vi "Configure Math (Add).vi"(0 "VISA resource name":refnum<visa-resource-name>, 2 "Vertical Scale (2)":dbl=2.0, 5 "Channel A (1: Channel 1)":i32(ring)=1 items=["Channel 1"=1, "Channel 2"=2, "Channel 3"=3, "Channel 4"=4], 7 "Channel B (2: Channel 2)":i32(ring)=2 items=["Channel 1"=1, "Channel 2"=2, "Channel 3"=3, "Channel 4"=4], 9 "Enable Invert Display (F: Disable)":bool, 11 "error in (no error)":errorcluster, 12 "Vertical Offset (0)":dbl) -> (4 "VISA resource name out":refnum<visa-resource-name>, 15 "error out":errorcluster)   [LabVIEW 2015, in "ZhiYuan ZDS Series for TCP.lvlib"]
doc: "Configures the setting for math operation with two operands."
uses:
  ZhiYuan ZDS Series for TCP.lvlib
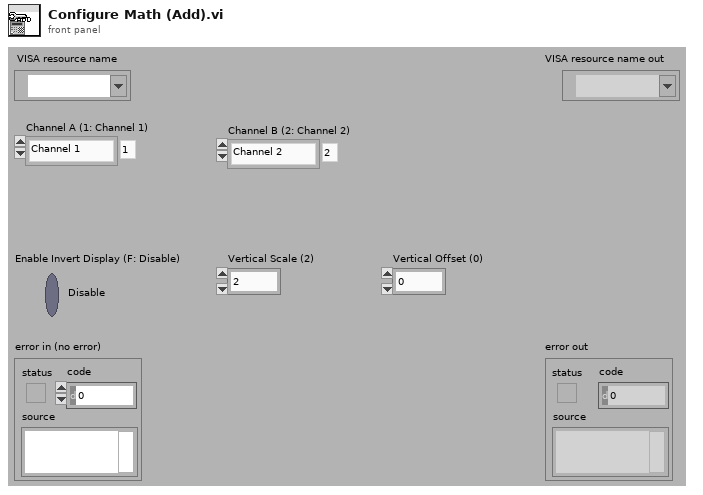
[diagram p1: front panel]
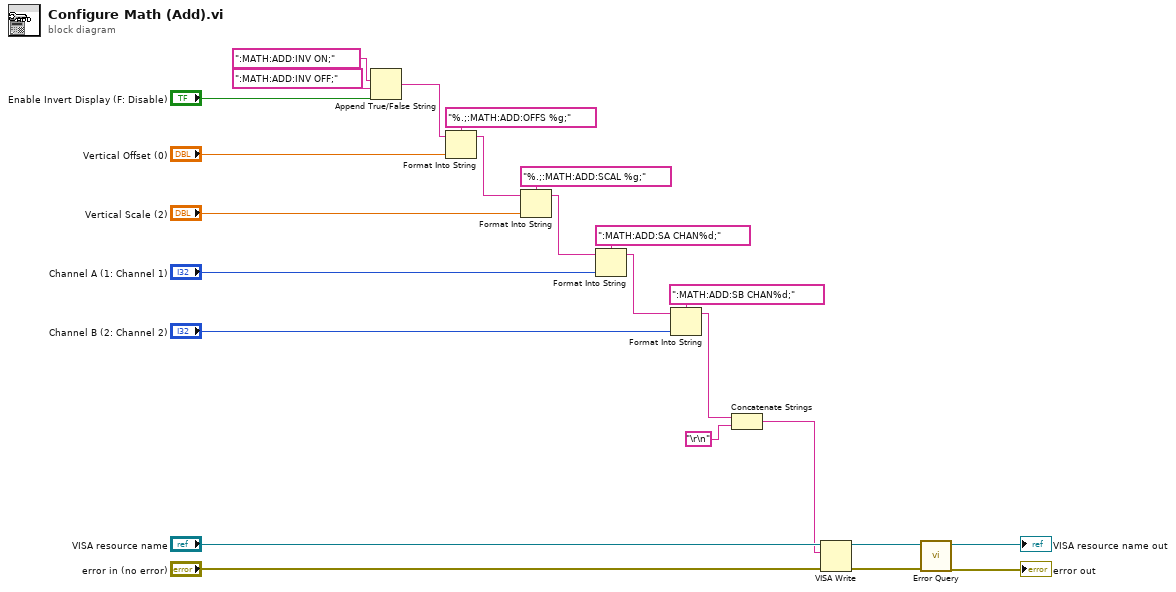
[diagram p0: block diagram]
diagram:
  n1 = Append True/False String(1:"Enable Invert Display (F: Disable)", 2:":MATH:ADD:INV OFF;", 3:":MATH:ADD:INV ON;") -> (0:w21:string)  [unwired: 1 in]
  n2 = Format Into String(format string="%.;:MATH:ADD:OFFS %g;", initial string=w21, "Vertical Offset (0)") -> (resulting string=w18:string)  [unwired: 1 in, 1 out]
  n3 = Format Into String(format string="%.;:MATH:ADD:SCAL %g;", initial string=w18, "Vertical Scale (2)") -> (resulting string=w15:string)  [unwired: 1 in, 1 out]
  n4 = Format Into String(format string=":MATH:ADD:SA CHAN%d;", initial string=w15, "Channel A (1: Channel 1)") -> (resulting string=w12:string)  [unwired: 1 in, 1 out]
  n5 = Format Into String(format string=":MATH:ADD:SB CHAN%d;", initial string=w12, "Channel B (2: Channel 2)") -> (resulting string=w3:string)  [unwired: 1 in, 1 out]
  n6 = Concatenate Strings(w3, "\r\n") -> (w1:string)
  n7 = VISA Write(VISA resource name="VISA resource name", write buffer=w1, error in (no error)="error in (no error)") -> (VISA resource name out=w7:refnum<visa-resource-name>, error out=w6:errorcluster)  [unwired: 1 out]
  n8 = call "Error Query.vi"("error in (no error)"=w6, "VISA resource name"=w7) -> ("error out"=→"error out":errorcluster, "VISA resource name out"=→"VISA resource name out":refnum<visa-resource-name>)  [unwired: 6 in, 2 out]
